vi "ADI_IMU_ADIS16470_Checksum.vi"(10 "Byte Array (MSB-First)":u8[](array[numeric])) -> (2 "Checksum":u16)   [LabVIEW 2017, in "ADIS16470_IMU.lvlib"]
uses:
  ADIS16470_IMU.lvlib
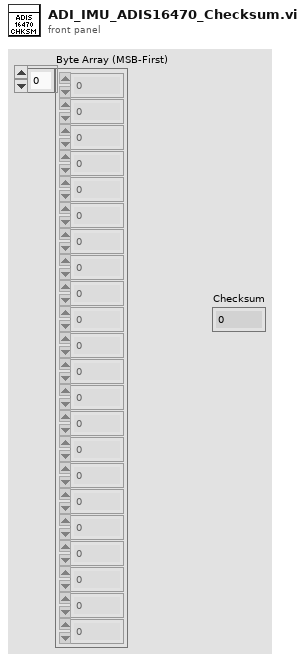
[diagram p1: front panel]
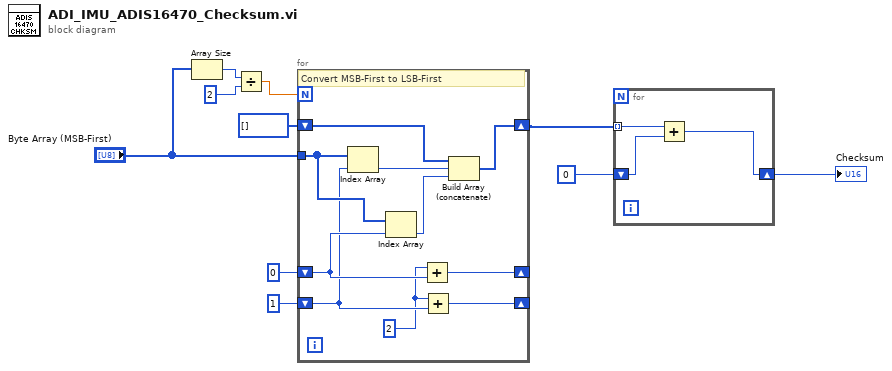
[diagram p0: block diagram]
diagram:
  n1 = Array Size(array="Byte Array (MSB-First)") -> (size(s)=w2:i32)
  n2 = Divide(x=w2, y=2) -> (x/y=w1:dbl)
  n3 = for {
    N: w1 -> [_]
    tunnel: "Byte Array (MSB-First)" -> [w20]
    shift-right: [w17] -> _
    shift-left: 0 -> [w19]
    shift-right: [w18] -> _
    shift-left: 1 -> [w16]
    shift-right: [w12] -> w9
    shift-left: u8[] [] -> [w11]
    w15 = 2 ("x")
    # "Convert MSB-First to LSB-First"
    n4 = Index Array(array=w20, index=w16) -> (element=w14:u8)
    n5 = Index Array(array=w20, index=w19) -> (element=w13:u8)
    n6 = Add(x=w15, y=w19) -> (x+y=w17:i32)
    n7 = Add(x=w15, y=w16) -> (x+y=w18:i32)
    n8 = Build Array (concatenate)(w11, w14, w13) -> (w12:u8[])
  }
  n9 = for {
    tunnel: w9 -> [w23] mode=indexing
    shift-right: [w21] -> w7
    shift-left: u16 0 -> [w22]
    n10 = Add(x=w23, y=w22) -> (x+y=w21:u16)
  }
  "Checksum" <- w7
